vi "E3_Write To Mesurement File.vi"() -> ()   [LabVIEW 2020]
uses:
  <vilib>/Analysis/NI_AALBase.lvlib
panel:
  out "Data":dbl(slide) scale=0.0..1.0
  out "mean":dbl format="%0.2f"
  out "min value":dbl
  out "max value":dbl
  out "Count":i32
  in  "stop":bool
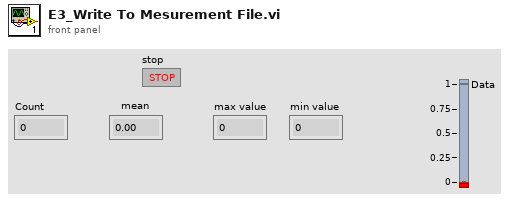
[diagram p1: front panel]
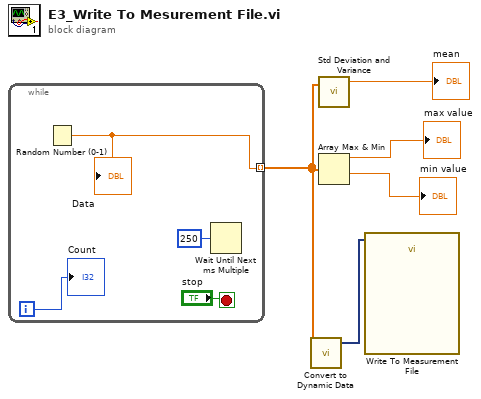
[diagram p0: block diagram]
diagram:
  n1 = while {
    tunnel: [w6] -> w1 mode=indexing
    i -> [w7]
    stop <- "stop" stop-if-true
    n2 = Random Number (0-1)() -> (number: 0 to 1=w6:dbl)
    "Data" <- w6
    n3 = Wait Until Next ms Multiple(millisecond multiple=u32 250) -> ()  [unwired: 1 out]
    "Count" <- w7
  }
  n4 = call "Convert to Dynamic Data"("Array"=w1) -> ("Dynamic Data Type"=w3:dynamicdata)  [unwired: 3 in]
  n5 = call <vilib>:"Std Deviation and Variance.vi"("X"=w1) -> ("mean"=→"mean":dbl)  [unwired: 1 in, 2 out]
  n6 = Array Max & Min(array=w1) -> (max value=→"max value":dbl, min value=→"min value":dbl)  [unwired: 2 out]
  n7 = call "Write To Measurement File"("Signals"=w3) -> ()  [unwired: 16 in, 3 out]
